vi "create GUID.vi"() -> (2 "GUID":T1 {"Lo" format="%.0x"; "Hi" format="%.0x"}, 3 "uuid":string)   [LabVIEW 2025, in "CEF.lvlib" / "CEF_serializable configuration.lvclass"]
doc: "Generates a unique identification stringCopyright 2017 National Instruments Corporation\n\nLicensed under the Apache License, Version 2.0 (the \"License\"); you may not use this file except in compliance with the License. You may obtain a copy of the License at http://www.apache.org/licenses/LICENSE-2.0\nUnless required by applicable law or agreed to in writing, software distributed under the License is distributed on an \"AS IS\" BASIS, WITHOUT WARRANTIES OR CONDITIONS OF ANY KIND, either express or implied. See the License for the specific language governing permissions and limitations under the License."
uses:
  CEF_serializable configuration.lvclass
  Numeric GUID.ctl
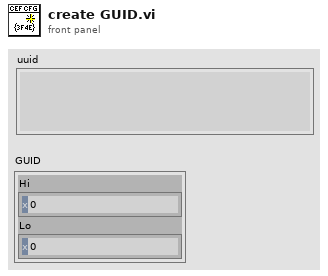
[diagram p1: front panel]
types:
  T1 = typedef "CEF.lvlib/CEF_serializable configuration.lvclass/Numeric GUID.ctl" = cluster{"Hi":u64, "Lo":u64}
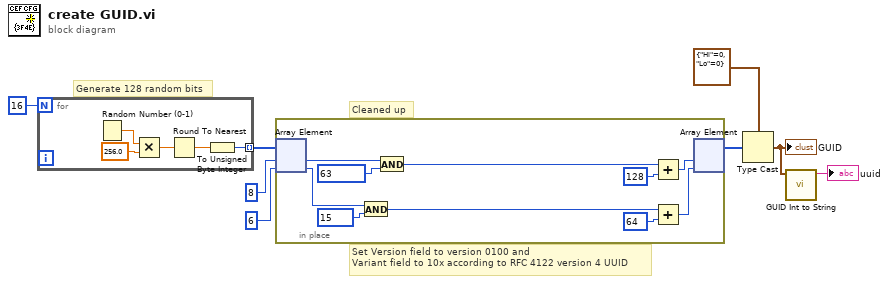
[diagram p0: block diagram]
diagram:
  # "Cleaned up"
  # "Set Version field to version 0100 and \nVariant field to 10x according to RFC 4122 version 4 UUID"
  # "Generate 128 random bits"
  n1 = for {
    N: 16 -> [_]
    tunnel: [w9] -> w7 mode=indexing
    n2 = Random Number (0-1)() -> (number: 0 to 1=w13:dbl)
    n3 = Multiply(x=w13, y=256.0) -> (x*y=w11:dbl)
    n4 = Round To Nearest(number=w11) -> (nearest integer value=w10:dbl)
    n5 = To Unsigned Byte Integer(number=w10) -> (unsigned 8bit integer=w9:u8)
  }
  n6 = in-place {
    n7 = in-place-array #1(w7, 8 ("index"), 6 ("index")) -> (w22:u8, w21:u8)
    n8 = And(x=w21, y=u8 15) -> (x .and. y?=w18:u8)
    n9 = And(x=w22, y=u8 63) -> (x .and. y?=w16:u8)
    n10 = Add(x=w16, y=u8 128) -> (x+y=w15:u8)
    n11 = Add(x=w18, y=u8 64) -> (x+y=w14:u8)
    n12 = in-place-array #1(w15, w14) -> (w3:u8[])  [unwired: 2 out]
  }
  n13 = Type Cast(type=T1 {"Hi"=0, "Lo"=0} ("GUID"), x=w3) -> (*(type *) &x=w1:T1)
  "GUID" <- w1
  n14 = call "GUID Int to String.vi"("GUID"=w1) -> ("uuid"=→"uuid":string)  [unwired: 10 in]
